vi "Write Realsense Cam.vi"(8 "error in (no error)":errorcluster, 10 "Realsense Cam.lvclass":refnum<class "Realsense Cam.lvclass">, 11 "Realsense Cam File Wrapper in":refnum<class "Realsense Cam File Wrapper.lvclass">) -> (0 "error out":errorcluster, 3 "Realsense Cam File Wrapper out":refnum<class "Realsense Cam File Wrapper.lvclass">)   [LabVIEW 2018, in "Realsense Cam File Wrapper.lvclass"]
uses:
  Realsense Cam File Wrapper.lvclass
  Realsense Cam/Realsense Cam.lvclass
  Realsense Cam File Wrapper.lvclass/Realsense Cam File Wrapper.ctl
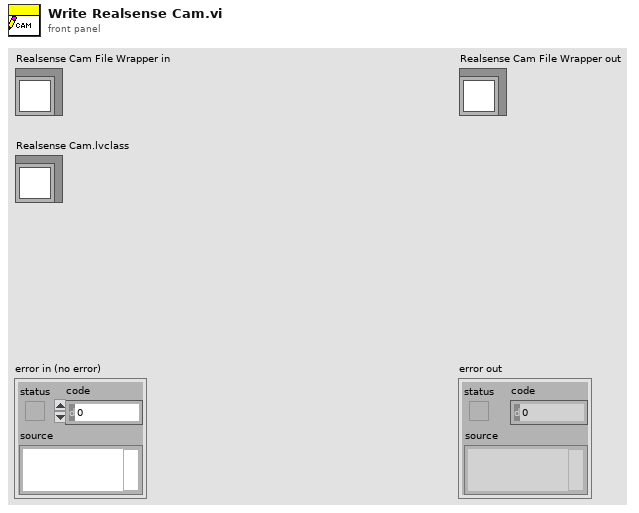
[diagram p1: front panel]
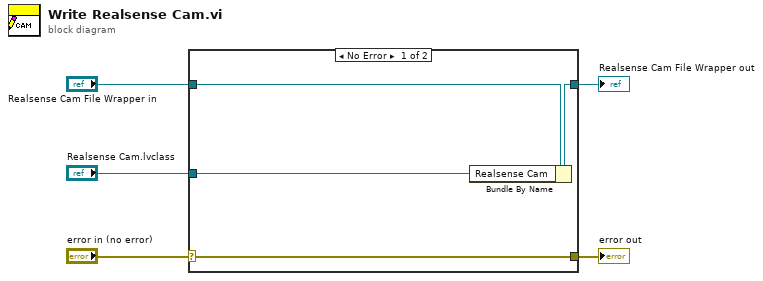
[diagram p0: block diagram]
diagram:
  n1 = case shown="No Error" "error in (no error)" {
    selector: "error in (no error)" -> [w9 w10]
    tunnel: [w9 w10] -> w4
    tunnel: [w7 w11] -> w2
    tunnel: "Realsense Cam File Wrapper in" -> [w8 w11]
    tunnel: "Realsense Cam.lvclass" -> [w6 _]
    frame No Error {
      n2 = Bundle By Name(cluster=w8, "Realsense Cam"=w6) -> (w7:refnum<class "Realsense Cam File Wrapper.lvclass">)
    }
    frame Error {
    }
  }
  "error out" <- w4
  "Realsense Cam File Wrapper out" <- w2
